vi "createEvents.vi"(8 "error in (no error)":errorcluster, 11 "SAL_Events in":refnum<class "SAL_Events.lvclass">) -> (0 "error out":errorcluster, 3 "SAL_Events out":refnum<class "SAL_Events.lvclass">)   [LabVIEW 2016, in "SAL_Events.lvclass"]
uses:
  SAL_Events.lvclass
  typedefs/eventsEvents.ctl
  SALLV_dome/DataTypes/logevent_AppliedSettingsMatchStart.ctl
  SALLV_dome/DataTypes/logevent_ErrorCode.ctl
  SALLV_dome/DataTypes/logevent_SettingVersions.ctl
  SALLV_dome/DataTypes/logevent_StateChanged.ctl
  SALLV_dome/DataTypes/logevent_SummaryState.ctl
  SAL_Events.lvclass/SAL_Events.ctl
  SALLV_dome/SALLV_dome.lvlib
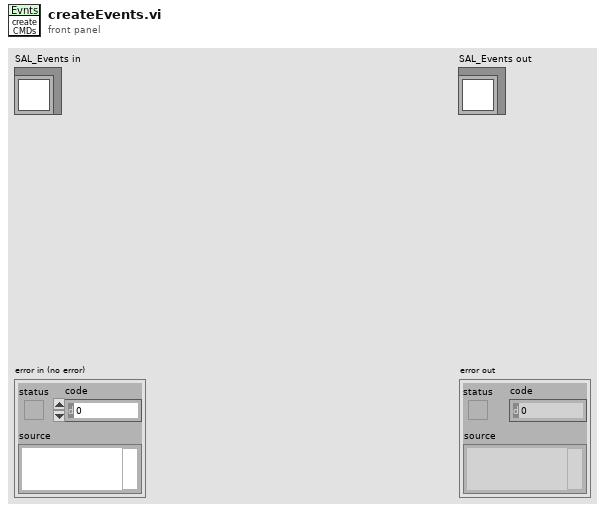
[diagram p1: front panel]
types:
  T1 = typedef "SALLV_dome.lvlib/logevent_AppliedSettingsMatchStart.ctl" = cluster{"appliedSettingsMatchStartIsTrue":bool, "priority":i32}
  T2 = typedef "SALLV_dome.lvlib/logevent_SummaryState.ctl" = cluster{"SummaryStateValue":enum16{"", "DisabledState", "EnabledState", "FaultState", "OfflineState", "StandbyState"}, "priority":i32}
  T3 = typedef "SALLV_dome.lvlib/logevent_StateChanged.ctl" = cluster{"newState":i32, "priority":i32}
  T4 = typedef "SALLV_dome.lvlib/logevent_SettingVersions.ctl" = cluster{"recommendedSettingVersion":string, "priority":i32}
  T5 = typedef "SALLV_dome.lvlib/logevent_ErrorCode.ctl" = cluster{"errorCode":i32, "priority":i32}
  T6 = typedef "eventsEvents.ctl" = cluster{"AppliedSettingsMatchStart":refnum<user-event>, "ErrorCode":refnum<user-event>, "SettingVersions":refnum<user-event>, "StateChanged":refnum<user-event>, "SummaryState":refnum<user-event>}
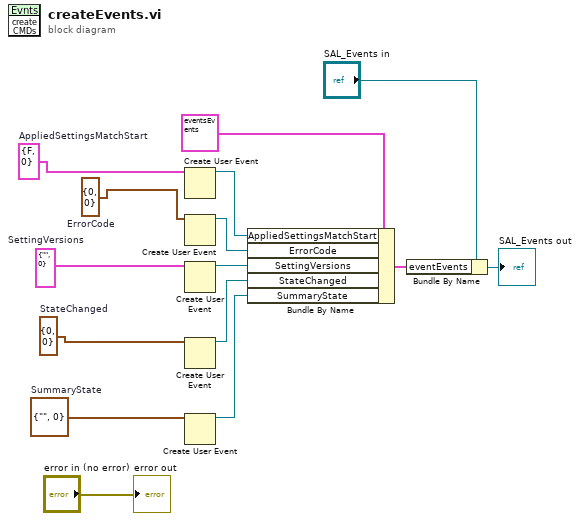
[diagram p0: block diagram]
diagram:
  w1 = T1 {"appliedSettingsMatchStartIsTrue"=FALSE, "priority"=0}  # AppliedSettingsMatchStart
  w5 = T2 {"SummaryStateValue"=enum."", "priority"=0}  # SummaryState
  w4 = T3 {"newState"=0, "priority"=0}  # StateChanged
  w3 = T4 {"recommendedSettingVersion"="", "priority"=0}  # SettingVersions
  w2 = T5 {"errorCode"=0, "priority"=0}  # ErrorCode
  n1 = Create User Event(user event datatype=w1) -> (user event=w10:refnum<user-event>)  [unwired: 1 in, 1 out]
  n2 = Create User Event(user event datatype=w2) -> (user event=w9:refnum<user-event>)  [unwired: 1 in, 1 out]
  n3 = Create User Event(user event datatype=w3) -> (user event=w8:refnum<user-event>)  [unwired: 1 in, 1 out]
  n4 = Create User Event(user event datatype=w4) -> (user event=w7:refnum<user-event>)  [unwired: 1 in, 1 out]
  n5 = Create User Event(user event datatype=w5) -> (user event=w6:refnum<user-event>)  [unwired: 1 in, 1 out]
  n6 = Bundle By Name(cluster=T6 {"AppliedSettingsMatchStart"=refnum, "ErrorCode"=refnum, "SettingVersions"=refnum, "StateChanged"=refnum, "SummaryState"=refnum} ("eventEvents"), "AppliedSettingsMatchStart"=w10, "ErrorCode"=w9, "SettingVersions"=w8, "StateChanged"=w7, "SummaryState"=w6) -> (w11:T6)
  n7 = Bundle By Name(cluster="SAL_Events in", "eventEvents"=w11) -> (→"SAL_Events out":refnum<class "SAL_Events.lvclass">)
  "error out" <- "error in (no error)"
